vi "switchCamera.vi"   [LabVIEW 2017]
uses:
  <vilib>/Rock Robotics/Network Tables/NT Write String.vi
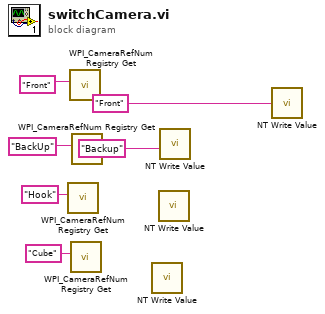
[diagram p0: block diagram]
diagram:
  n1 = call <vilib>:"WPI_CameraRefNum Registry Get.vi"("refnum name"="Hook") -> ()  [unwired: 9 in, 2 out]
  n2 = call <vilib>:"WPI_CameraRefNum Registry Get.vi"("refnum name"="Front") -> ()  [unwired: 9 in, 2 out]
  n3 = call <vilib>:"WPI_CameraRefNum Registry Get.vi"("refnum name"="Cube") -> ()  [unwired: 9 in, 2 out]
  n4 = call <vilib>:"WPI_CameraRefNum Registry Get.vi"("refnum name"="BackUp") -> ()  [unwired: 9 in, 2 out]
  n5 = call-poly <vilib>:"NT Write Value.vi"() -> ()  [unwired: 11 in, 1 out]
  n6 = call-poly <vilib>:"NT Write Value.vi"() -> ()  [unwired: 11 in, 1 out]
  n7 = call-poly <vilib>:"NT Write Value.vi"("String"="Backup") -> ()  [unwired: 10 in, 1 out]
  n8 = call-poly <vilib>:"NT Write Value.vi"("Name"="Front") -> ()  [unwired: 10 in, 1 out]
